vi "Get Chamber Status.vi"(8 "error in (no error)":errorcluster) -> (0 "error out":errorcluster)   [LabVIEW 2018]
uses:
  <vilib>/addons/_JKI Toolkits/Caraya/classes/Test/Test.lvclass
  Libraries/Thermal Chamber Response Simulator/Thermal Chamber Response Simulator.lvlib
  <vilib>/addons/_JKI Toolkits/Caraya/classes/Assert/Assert.lvclass
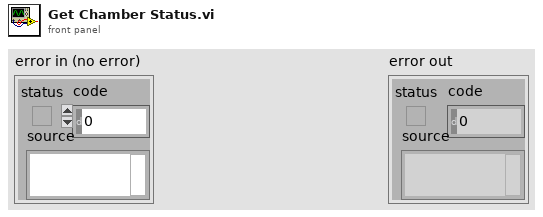
[diagram p1: front panel]
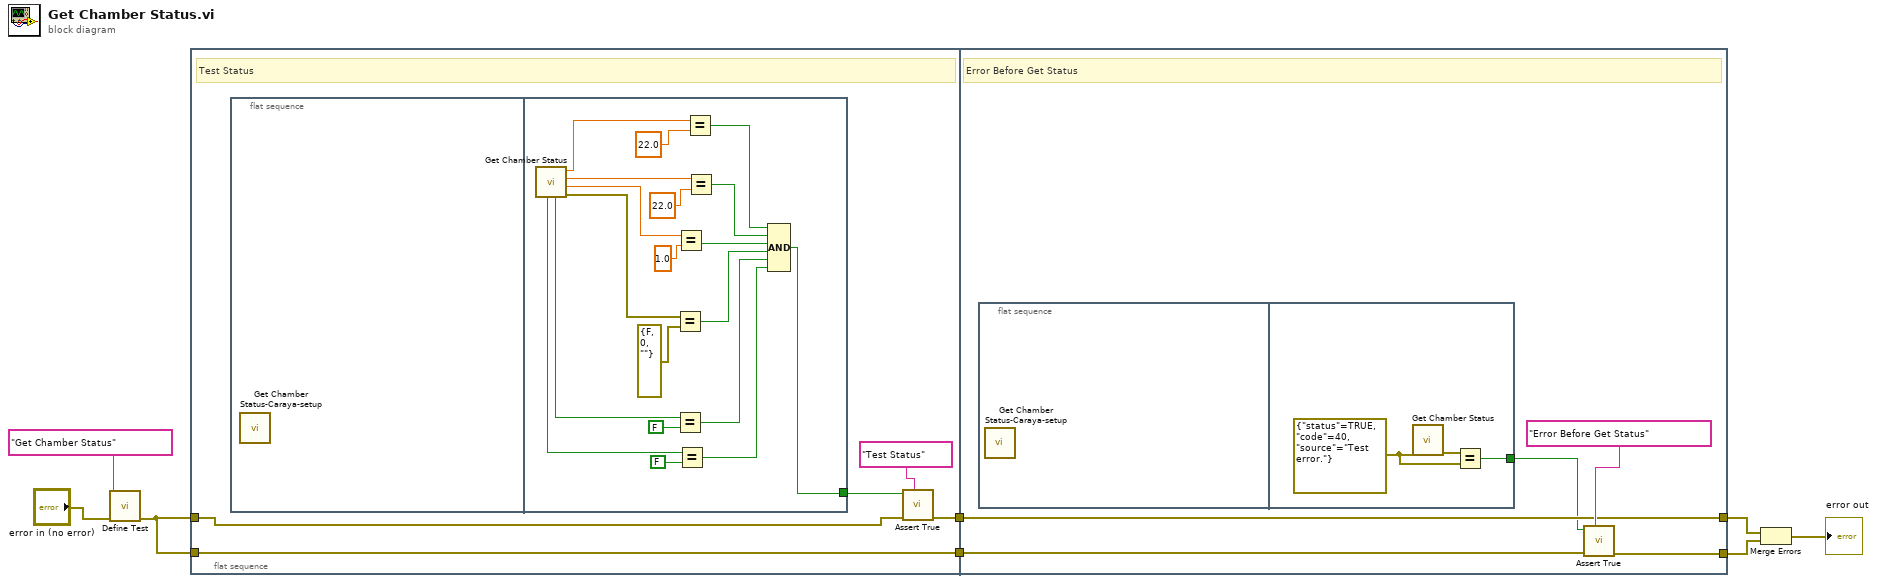
[diagram p0: block diagram]
diagram:
  n1 = call <vilib>:"Define Test.vi"("error in (no error)"="error in (no error)", "Label (VI Title)"="Get Chamber Status") -> ("error out"=w6:errorcluster)  [unwired: 9 in]
  n2 = flat-sequence {
    tunnel: w6 -> [w9]
    tunnel: [w12] -> w7
    tunnel: w6 -> [w11]
    tunnel: [w11] -> w5
    tunnel: w7 -> [w35]
    tunnel: [w36] -> w4
    tunnel: [w35] -> w3
    tunnel: w5 -> [w34]
    frame #0 {
      # "Test Status"
      n3 = flat-sequence {
        tunnel: [w14] -> w10
        frame #0 {
          n4 = call "Get Chamber Status-Caraya-setup.vi"() -> ()  [unwired: 12 in]
        }
        frame #1 {
          n5 = call "Get Chamber Status.vi"() -> ("error out"=w29:errorcluster, "Ramp Rate (deg C / second)"=w30:dbl, "Temperature Set Point (deg C)"=w31:dbl, "Actual Temperature"=w32:dbl, "Application Exit"=w28:bool, "Heater State"=w27:bool)  [unwired: 6 in]
          n6 = Equal?(x=w29, y=errorcluster {"status"=FALSE, "code"=0, "source"=""}) -> (x = y?=w17:bool)
          n7 = Equal?(x=w28, y=FALSE) -> (x = y?=w16:bool)
          n8 = Equal?(x=w30, y=1.0) -> (x = y?=w18:bool)
          n9 = Equal?(x=w27, y=FALSE) -> (x = y?=w15:bool)
          n10 = Equal?(x=w32, y=22.0) -> (x = y?=w20:bool)
          n11 = Equal?(x=w31, y=22.0) -> (x = y?=w19:bool)
          n12 = Compound Arithmetic op=AND(w20, w19, w18, w17, w16, w15) -> (w14:bool)
        }
      }
      n13 = call <vilib>:"Assert True.vi"("Label"="Test Status", "error in (no error)"=w9, "True?"=w10) -> ("error out"=w12:errorcluster)  [unwired: 8 in]
    }
    frame #1 {
      # "Error Before Get Status"
      n14 = flat-sequence {
        tunnel: [w38] -> w33
        frame #0 {
          n15 = call "Get Chamber Status-Caraya-setup.vi"() -> ()  [unwired: 12 in]
        }
        frame #1 {
          w39 = errorcluster {"status"=TRUE, "code"=40, "source"="Test error."} ("Test Error")
          n16 = call "Get Chamber Status.vi"("error in (no error)"=w39) -> ("error out"=w40:errorcluster)  [unwired: 5 in, 5 out]
          n17 = Equal?(x=w40, y=w39) -> (x = y?=w38:bool)
        }
      }
      n18 = call <vilib>:"Assert True.vi"("Label"="Error Before Get Status", "error in (no error)"=w34, "True?"=w33) -> ("error out"=w36:errorcluster)  [unwired: 8 in]
    }
  }
  n19 = Merge Errors(w3, w4) -> (→"error out":errorcluster)
